vi "Insert Bound View.vi"(8 "error in (no error)":errorcluster, 9 "Value Publication Time":timestamp, 10 "Selector Value":string, 11 "BoundViewManager in":refnum<class "BoundViewManager.lvclass">) -> (0 "error out":errorcluster, 3 "BoundViewManager out":refnum<class "BoundViewManager.lvclass">)   [LabVIEW 2017, in "BoundViewManager.lvlib" / "BoundViewManager.lvclass"]
uses:
  BoundViewManager.lvclass
  <vilib>/ActorFramework/Message Enqueuer/Message Enqueuer.lvclass
  BoundViewManager.lvclass/BoundViewManager.ctl
  Framework/IViewable/IViewable Messages/Insert Front Panel Msg/Insert Front Panel Msg.lvclass/Insert Front Panel Msg.ctl
  <vilib>/ActorFramework/Message Enqueuer/Message Enqueuer.lvclass/Message Enqueuer.ctl
  <vilib>/ActorFramework/Message Enqueuer/Enqueue.vi
  Framework/IViewable/IViewable Messages/Insert Front Panel Msg/Insert Front Panel Msg.lvclass
  C:/Program Files (x86)/National Instruments/LabVIEW 2017/vi.lib/ActorFramework/Message/Message.lvclass
  <vilib>/ActorFramework/Message Priority Queue/Priority Enqueue.vi
  <vilib>/Composed Systems/Current Value Table/CurrentValueTable.lvclass
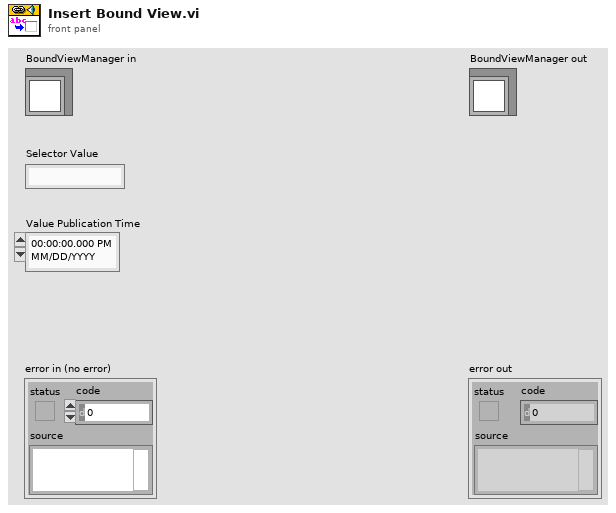
[diagram p1: front panel]
types:
  T1 = typedef "CurrentValueTable.lvlib/CurrentValueTable.lvclass/CurrentValueTable Reference.ctl" = refnum<data-value>
  T2 = typedef "IViewable.lvlib/ProtectedSubpanel.lvclass/Protected Subpanel Reference.ctl" = refnum<data-value>
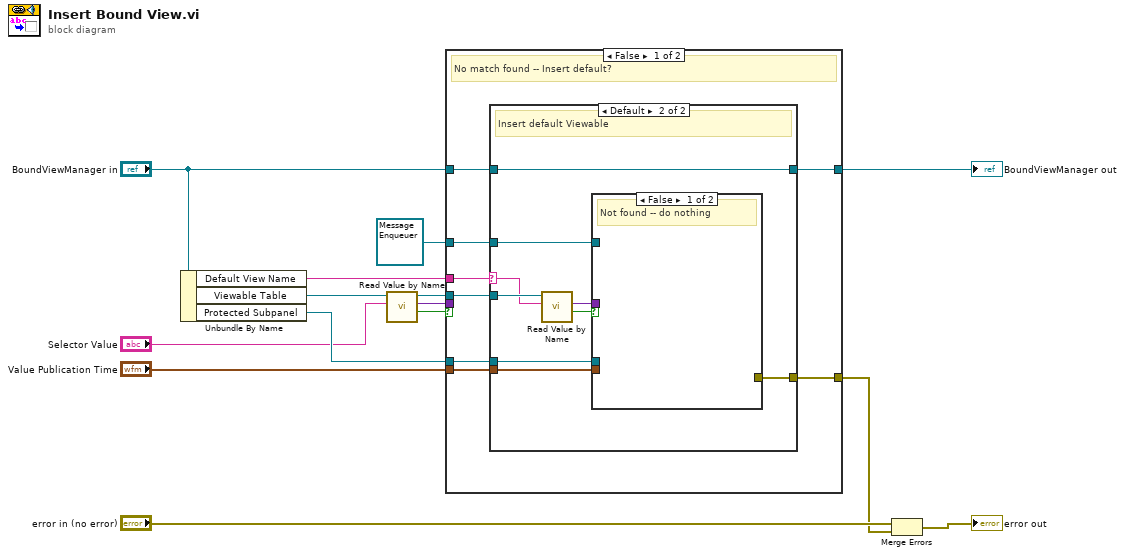
[diagram p0: block diagram]
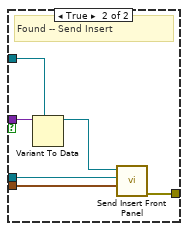
[diagram p3: hidden frame]
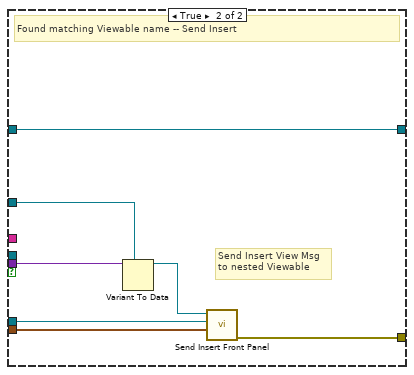
[diagram p4: hidden frame]
diagram:
  n1 = Unbundle By Name("BoundViewManager in") -> ("Default View Name"=w4:string, "Viewable Table"=w13:T1, "Protected Subpanel"=w12:T2)
  n2 = call <vilib>:"Read Value by Name.vi"("Data Name"="Selector Value", "Current Value Table"=w13) -> ("Value Found?"=w9:bool, "Current Value"=w11:variant, "Current Value Table"=w2:T1)  [unwired: 6 in, 1 out]
  n3 = case shown="False" w9 {
    tunnel: w12 -> [w19 w45]
    tunnel: w11 -> [_ w44]
    tunnel: "Value Publication Time" -> [w18 w42]
    tunnel: [w17 w41] -> w7
    tunnel: "BoundViewManager in" -> [w22 w40]
    tunnel: [w21 w40] -> w5
    tunnel: w4 -> [w20 _]
    tunnel: w2 -> [w16 _]
    tunnel: refnum<class "Message Enqueuer.lvclass"> refnum ("Message Enqueuer") -> [w15 w39]
    frame False {
      # "No match found -- Insert default?"
      n4 = case shown="Default" w20 {
        selector: w20 -> [_ w27]
        tunnel: w22 -> [w23 w29]
        tunnel: [w23 w29] -> w21
        tunnel: w19 -> [_ w32]
        tunnel: w18 -> [_ w31]
        tunnel: [_ w30] -> w17
        tunnel: w16 -> [_ w28]
        tunnel: w15 -> [_ w25]
        frame "" {
          # "No default set -- No Viewable state change"
        }
        frame Default {
          # "Insert default Viewable"
          n5 = call <vilib>:"Read Value by Name.vi"("Data Name"=w27, "Current Value Table"=w28) -> ("Value Found?"=w24:bool, "Current Value"=w26:variant)  [unwired: 6 in, 2 out]
          n6 = case shown="False" w24 {
            tunnel: w32 -> [_ w38]
            tunnel: w31 -> [_ w37]
            tunnel: [_ w36] -> w30
            tunnel: w26 -> [_ w35]
            tunnel: w25 -> [_ w34]
            frame False {
              # "Not found -- do nothing"
            }
            frame True {
              # "Found -- Send Insert"
              n7 = Variant To Data(type=w34, Variant=w35) -> (data=w33:refnum<class "Message Enqueuer.lvclass">)  [unwired: 1 in, 1 out]
              n8 = call "Send Insert Front Panel.vi"("Request Time"=w37, "Protected Subpanel"=w38, "Message Enqueuer"=w33) -> ("error out"=w36:errorcluster)  [unwired: 7 in, 1 out]
            }
          }
        }
      }
    }
    frame True {
      # "Send Insert View Msg\nto nested Viewable"
      # "Found matching Viewable name -- Send Insert"
      n9 = Variant To Data(type=w39, Variant=w44) -> (data=w43:refnum<class "Message Enqueuer.lvclass">)  [unwired: 1 in, 1 out]
      n10 = call "Send Insert Front Panel.vi"("Request Time"=w42, "Protected Subpanel"=w45, "Message Enqueuer"=w43) -> ("error out"=w41:errorcluster)  [unwired: 7 in, 1 out]
    }
  }
  "BoundViewManager out" <- w5
  n11 = Merge Errors("error in (no error)", w7) -> (→"error out":errorcluster)
